vi "Drive distance with time1.vi"(8 "error in (no error)":errorcluster, 11 "Wanted Distance":dbl) -> (0 "error out":errorcluster)   [LabVIEW 2017]
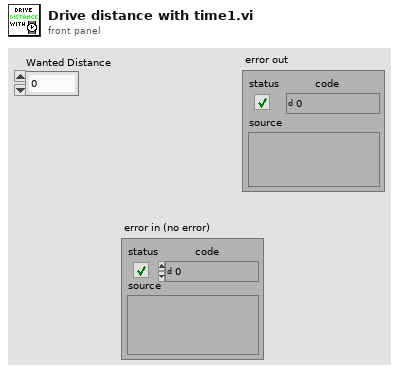
[diagram p1: front panel]
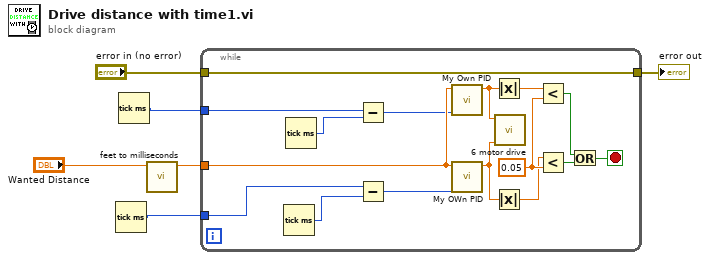
[diagram p0: block diagram]
diagram:
  n1 = Tick Count (ms)() -> (millisecond timer value=w2:u32)
  n2 = Tick Count (ms)() -> (millisecond timer value=w1:u32)
  n3 = call "feet to milliseconds.vi"("Distance in feet wanted"="Wanted Distance") -> ("milliseconds"=w5:dbl)  [unwired: 10 in]
  n4 = while {
    tunnel: w5 -> [w22]
    tunnel: [w17] -> w4
    tunnel: "error in (no error)" -> [w17]
    tunnel: w1 -> [w8]
    tunnel: w2 -> [w9]
    stop <- w21 stop-if-true
    w20 = 0.05
    n5 = Tick Count (ms)() -> (millisecond timer value=w10:u32)
    n6 = Tick Count (ms)() -> (millisecond timer value=w7:u32)
    n7 = Subtract(x=w8, y=w7) -> (x-y=w12:u32)
    n8 = Subtract(x=w9, y=w10) -> (x-y=w11:u32)
    n9 = call "My Own PID.vi"("Current Input"=w12, "Wanted End"=w22) -> ("Output"=w14:dbl)  [unwired: 9 in]
    n10 = call "My OWn PID.vi"("Current Input"=w11, "Wanted End"=w22) -> ("Output"=w16:dbl)  [unwired: 9 in]
    n11 = Absolute Value(x=w14) -> (abs(x)=w13:dbl)
    n12 = Absolute Value(x=w16) -> (abs(x)=w15:dbl)
    n13 = call "6 motor drive.vi"("Right Joystick"=w16, "Left Joystick"=w14) -> ()  [unwired: 10 in]
    n14 = Less?(x=w13, y=w20) -> (x < y?=w19:bool)
    n15 = Less?(x=w15, y=w20) -> (x < y?=w18:bool)
    n16 = Or(x=w19, y=w18) -> (x .or. y?=w21:bool)
  }
  "error out" <- w4
